vi "RequestInsertObj.vi"(5 "Array":T1[](array[typedef]), 11 "error in (no error)":errorcluster) -> (6 "request":string, 15 "error out":errorcluster)   [LabVIEW 2019, in "Logger.lvclass"]
uses:
  Logger.lvclass
  ObjData.ctl
  ObjType.ctl
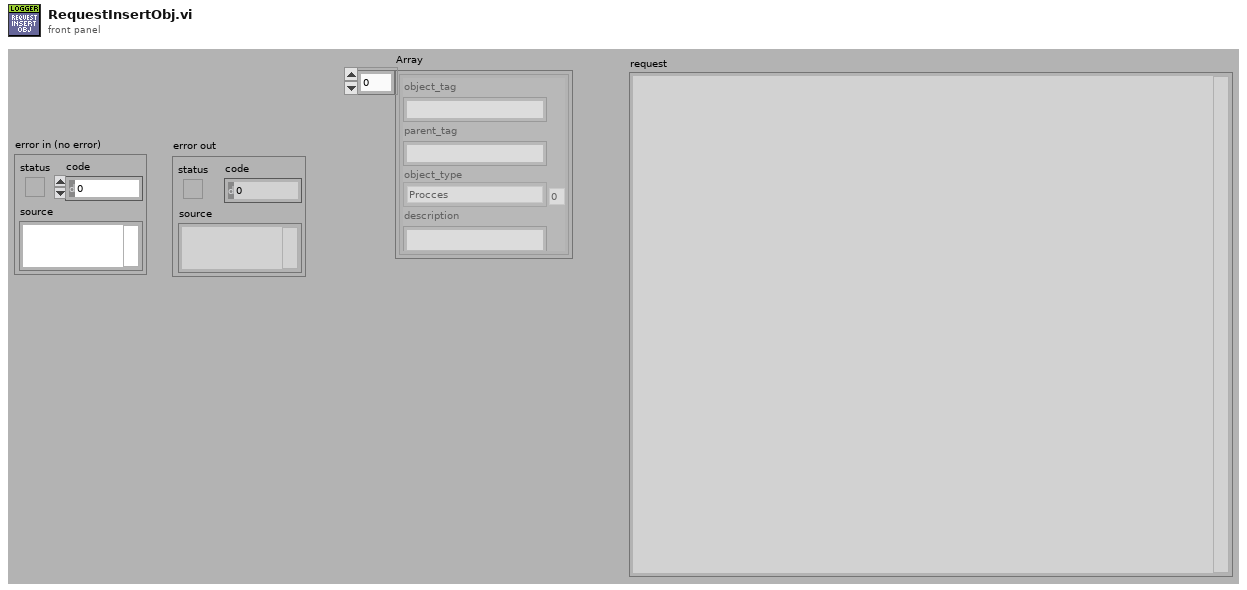
[diagram p1: front panel]
types:
  T1 = typedef "Logger.lvclass/ObjData.ctl" = cluster{"object_tag":string, "parent_tag":string, "object_type":T2, "description":string}
  T2 = typedef "Logger.lvclass/ObjType.ctl" = enum16{"Procces", "Device", "SignalA", "SignalD", "DI", "DO", "DA", "AI", "AO", "AA", "GUI"}
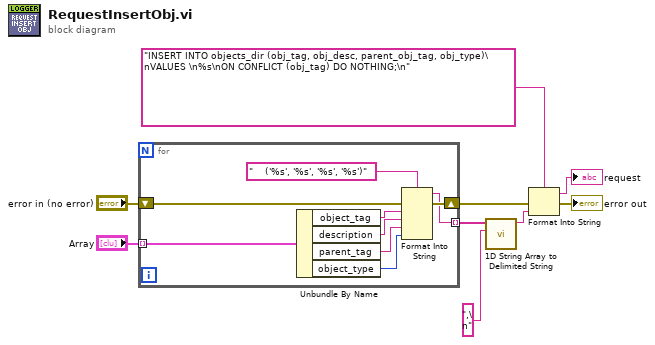
[diagram p0: block diagram]
diagram:
  n1 = for {
    tunnel: [w17] -> w8 mode=indexing
    tunnel: "Array" -> [w16] mode=indexing
    shift-right: [w18] -> w3
    shift-left: "error in (no error)" -> [w15]
    n2 = Unbundle By Name(w16) -> ("object_tag"=w13:string, "description"=w12:string, "parent_tag"=w11:string, "object_type"=w10:T2)
    n3 = Format Into String(format string="    ('%s', '%s', '%s', '%s')", error in=w15, w13, w12, w11, w10) -> (resulting string=w17:string, error out=w18:errorcluster)  [unwired: 1 in]
  }
  n4 = call <vilib>:"1D String Array to Delimited String.vi"("delimiter"=",\n", "string array"=w8) -> ("delimited string"=w4:string)  [unwired: 9 in]
  n5 = Format Into String(format string="INSERT INTO objects_dir (obj_tag, obj_desc, parent_obj_tag, obj_type)\nVALUES \n%s\nON CONFLICT (obj_tag) DO NOTHING;\n", error in=w3, w4) -> (resulting string=→"request":string, error out=→"error out":errorcluster)  [unwired: 1 in]
